vi "FeedbackDecode_ParsePickROIStr.vi"(0 "Perception_array":string[](array[string]), 1 "Description_array":string[](array[string]), 2 "X_array":dbl[][](array[numeric]), 3 "Y_array":dbl[][](array[numeric]), 4 "Sensor_array":string[][](array[string]), 5 "Region_array":string[][](array[string])) -> (16 "ROIStr":string)   [LabVIEW 2020]
panel:
  out "SensationStr":string
  out "DescStr":string
  out "RegionStr":string
  out "SensorStr":string
  out "LocationStr":string
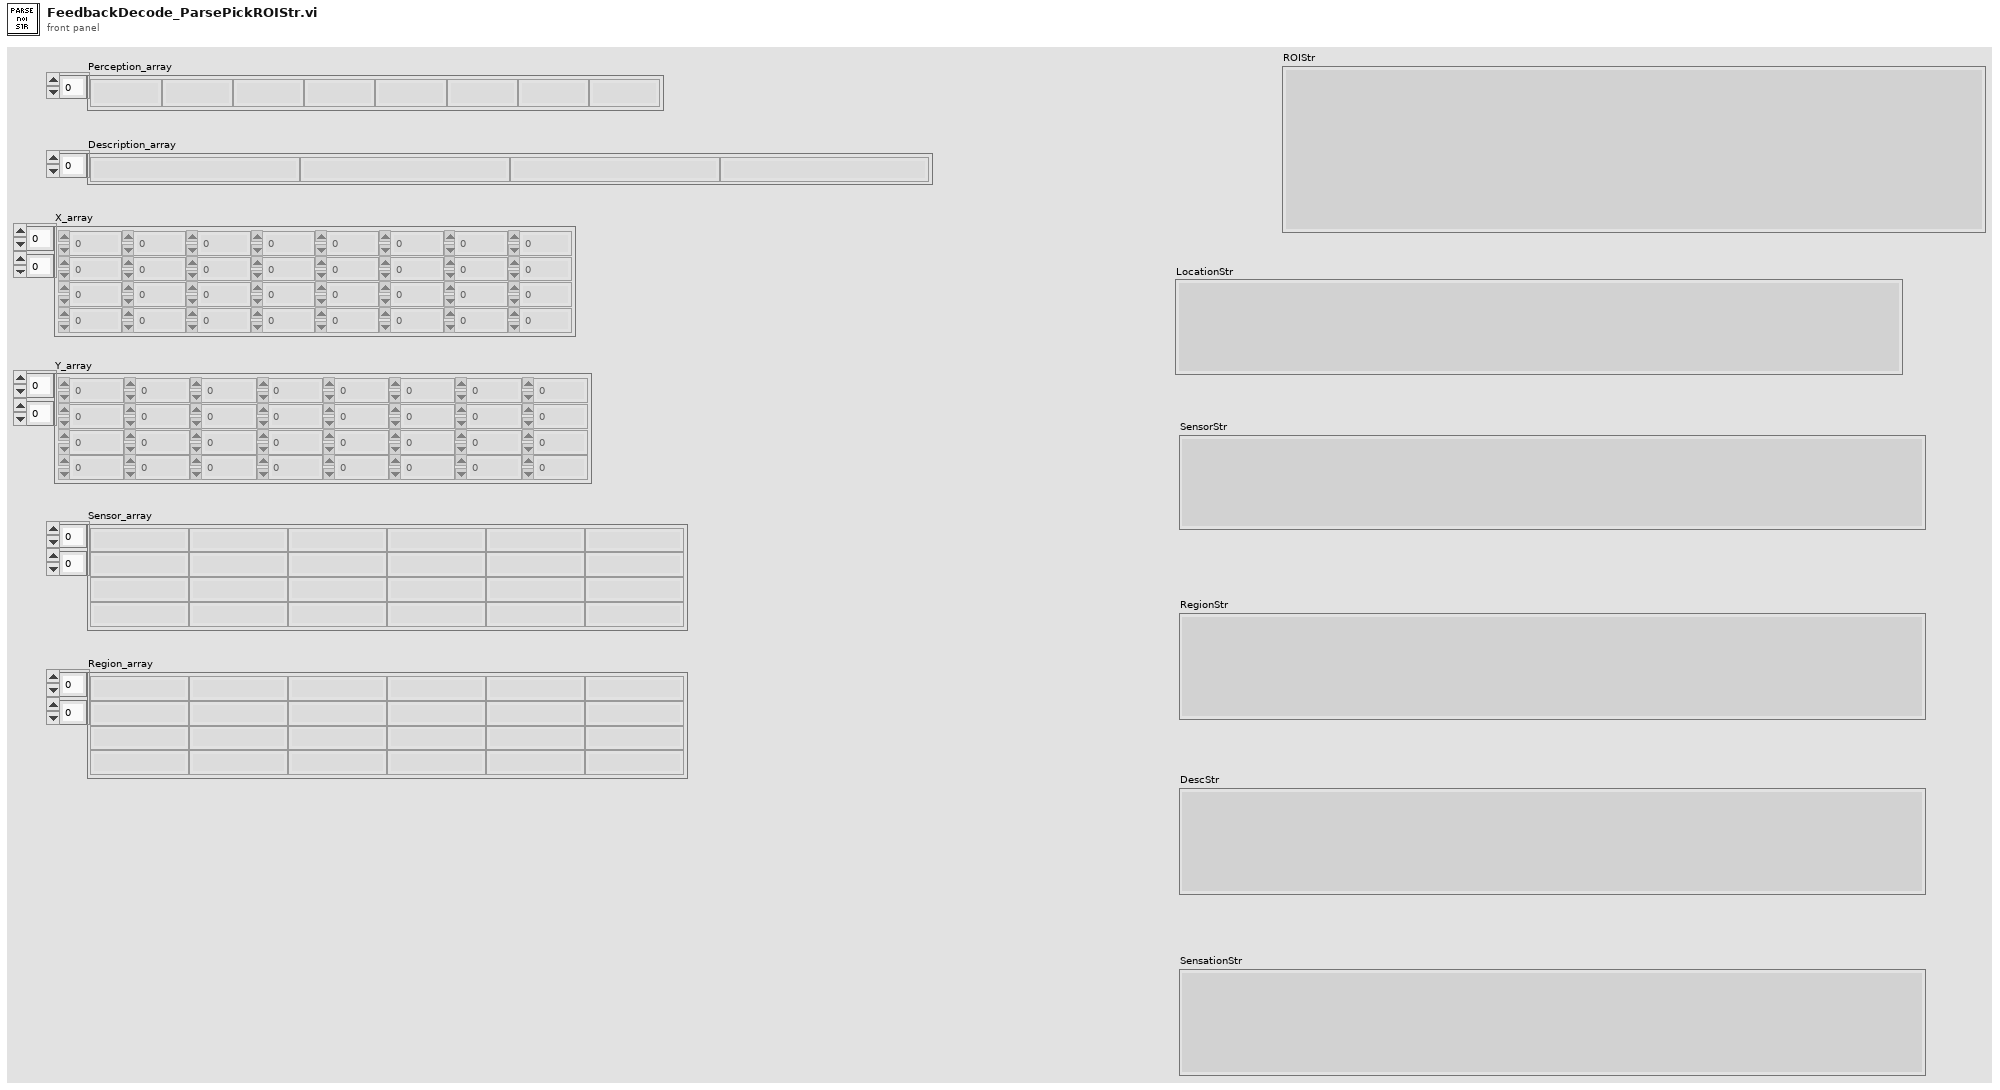
[diagram p1: front panel]
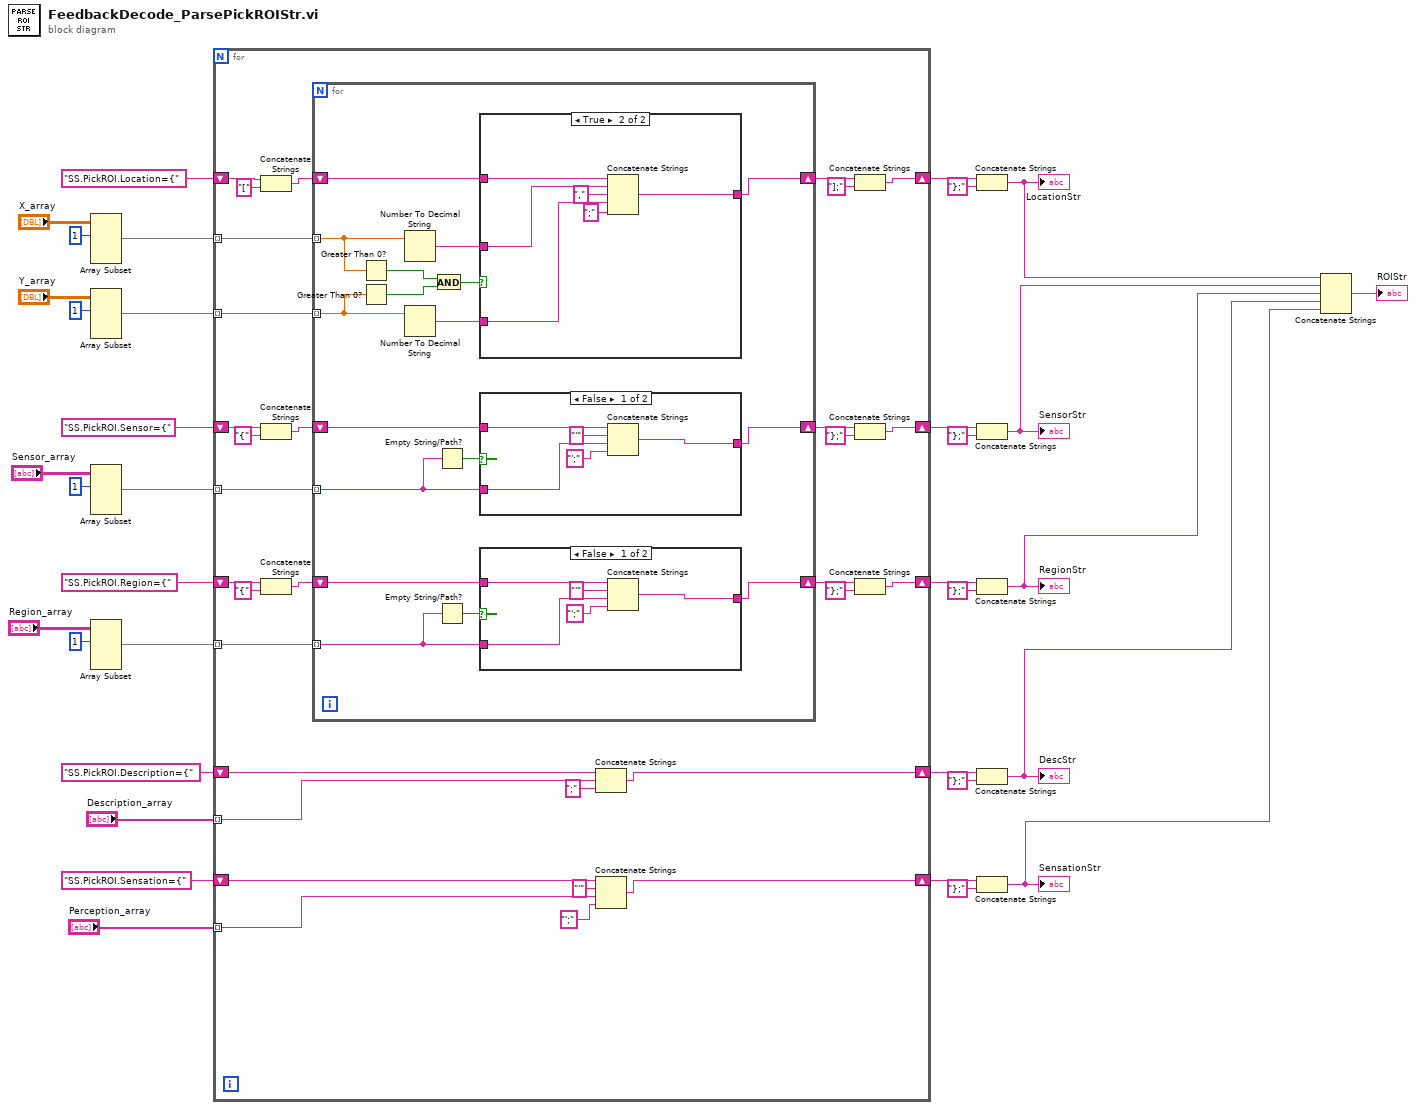
[diagram p0: block diagram]
diagram:
  n1 = Array Subset(array="X_array", index (row)=1 ("index")) -> (w31:dbl[][])  [unwired: 3 in]
  n2 = Array Subset(array="Y_array", index (row)=1 ("index")) -> (w30:dbl[][])  [unwired: 3 in]
  n3 = Array Subset(array="Sensor_array", index (row)=1 ("index")) -> (w23:string[][])  [unwired: 3 in]
  n4 = Array Subset(array="Region_array", index (row)=1 ("index")) -> (w18:string[][])  [unwired: 3 in]
  n5 = for {
    tunnel: w31 -> [w66] mode=indexing
    tunnel: w30 -> [w65] mode=indexing
    shift-right: [w59] -> w27
    shift-left: "SS.PickROI.Location={" -> [w64]
    shift-right: [w52] -> w21
    shift-left: "SS.PickROI.Sensor={" -> [w56]
    tunnel: w23 -> [w58] mode=indexing
    shift-right: [w51] -> w20
    shift-left: "SS.PickROI.Region={" -> [w47]
    tunnel: w18 -> [w45] mode=indexing
    tunnel: "Description_array" -> [w42] mode=indexing
    shift-right: [w41] -> w11
    shift-left: "SS.PickROI.Description={" -> [w43]
    tunnel: "Perception_array" -> [w39] mode=indexing
    shift-right: [w40] -> w10
    shift-left: "SS.PickROI.Sensation={" -> [w38]
    n6 = Concatenate Strings(w64, "[" ("string")) -> (w62:string)
    n7 = Concatenate Strings(w56, "{" ("string")) -> (w55:string)
    n8 = Concatenate Strings(w47, "{" ("string")) -> (w48:string)
    n9 = for {
      tunnel: w66 -> [w83] mode=indexing
      tunnel: w65 -> [w82] mode=indexing
      shift-right: [w75] -> w60
      shift-left: w62 -> [w78]
      shift-right: [w73] -> w53
      shift-left: w55 -> [w74]
      tunnel: w58 -> [w71] mode=indexing
      shift-right: [w68] -> w50
      shift-left: w48 -> [w67]
      tunnel: w45 -> [w70] mode=indexing
      n10 = Greater Than 0?(x=w83) -> (x > 0?=w81:bool)
      n11 = Greater Than 0?(x=w82) -> (x > 0?=w80:bool)
      n12 = Number To Decimal String(number=w83) -> (decimal integer string=w77:string)  [unwired: 1 in]
      n13 = Number To Decimal String(number=w82) -> (decimal integer string=w76:string)  [unwired: 1 in]
      n14 = And(x=w81, y=w80) -> (x .and. y?=w79:bool)
      n15 = Empty String/Path?(string/path=w71) -> (empty?=w72:bool)
      n16 = Empty String/Path?(string/path=w70) -> (empty?=w69:bool)
      n17 = case shown="True" w79 {
        tunnel: w78 -> [w96 w102]
        tunnel: w77 -> [_ w101]
        tunnel: w76 -> [_ w99]
        tunnel: [w96 w97] -> w75
        frame False {
        }
        frame True {
          n18 = Concatenate Strings(w102, w101, "," ("string"), w99, ";" ("string")) -> (w97:string)
        }
      }
      n19 = case shown="False" w72 {
        tunnel: [w92 w95] -> w73
        tunnel: w74 -> [w91 w95]
        tunnel: w71 -> [w90 _]
        frame False {
          n20 = Concatenate Strings(w91, "'" ("string"), w90, "';" ("string")) -> (w92:string)
        }
        frame True {
        }
      }
      n21 = case shown="False" w69 {
        tunnel: [w86 w89] -> w68
        tunnel: w67 -> [w85 w89]
        tunnel: w70 -> [w84 _]
        frame False {
          n22 = Concatenate Strings(w85, "'" ("string"), w84, "';" ("string")) -> (w86:string)
        }
        frame True {
        }
      }
    }
    n23 = Concatenate Strings(w43, w42, ";" ("string")) -> (w41:string)
    n24 = Concatenate Strings(w38, "'" ("string"), w39, "';" ("string")) -> (w40:string)
    n25 = Concatenate Strings(w60, "];" ("string")) -> (w59:string)
    n26 = Concatenate Strings(w53, "};" ("string")) -> (w52:string)
    n27 = Concatenate Strings(w50, "};" ("string")) -> (w51:string)
  }
  n28 = Concatenate Strings(w27, "};" ("string")) -> (w6:string)
  "LocationStr" <- w6
  n29 = Concatenate Strings(w21, "};" ("string")) -> (w5:string)
  "SensorStr" <- w5
  n30 = Concatenate Strings(w20, "};" ("string")) -> (w4:string)
  "RegionStr" <- w4
  n31 = Concatenate Strings(w11, "};" ("string")) -> (w3:string)
  "DescStr" <- w3
  n32 = Concatenate Strings(w10, "};" ("string")) -> (w2:string)
  "SensationStr" <- w2
  n33 = Concatenate Strings(w6, w5, w4, w3, w2) -> (→"ROIStr":string)
